vi "Stream.vi"(0 "reference in":refnum<class "Streamer.lvclass">, 5 "error in":errorcluster) -> (14 "reference out":refnum<class "Streamer.lvclass">, 19 "error out":errorcluster)   [LabVIEW 2023, in "Streamer.lvclass"]
uses:
  Streamer.lvclass
  <instrlib>/HPS-17000/HPS-17000.lvclass
  <vilib>/HPS-17000/MStream_grpc_CyclerMeasurement.ctl
  Streamer.lvclass/Streamer.ctl
  <vilib>/Utility/SystemLogging/NI_SystemLogging.lvlib
  <vilib>/HPS-17000/NI_BC_client.lvlib
panel:
  out "error info":errorcluster
  out "Last Command":string
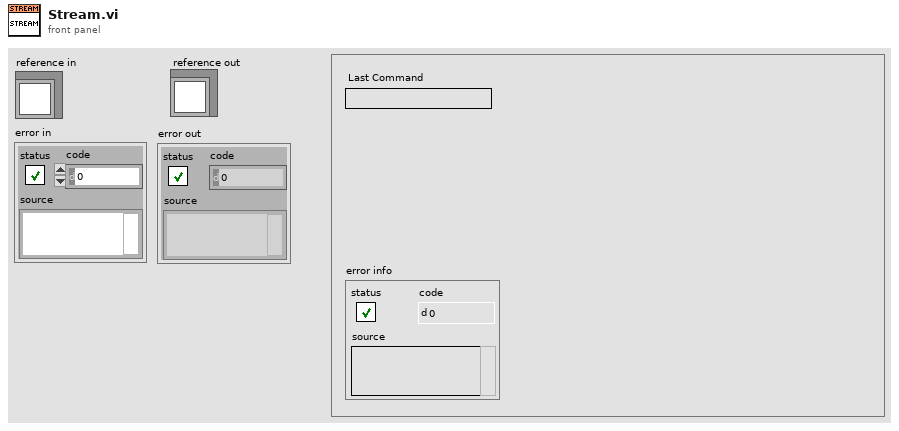
[diagram p1: front panel]
types:
  T1 = cluster{"Core":cluster{"Timeout":i32, "Events":cluster{"EventsToProcess":refnum<event-registration>}, "EventFromProcess":refnum<user-event>, "ProcessSyncQueue":refnum<queue>, "QueueFromProcess":refnum<queue>, "Command":string, "Data":variant}, "HPS17K Refs":refnum<class "HPS-17000.lvclass">[], "Stream Queues":refnum<queue>[]}
  T2 = enum32{"Invalid", "Standard", "Closed", "Hidden", "Minimized", "Maximized"}
  T3 = cluster{"EventsToProcess":refnum<event-registration>}
  T4 = typedef "NI_BC_client.lvlib/MStream_grpc_CyclerMeasurement.ctl" = cluster{"measured_voltage":sgl, "measured_current":sgl, "setpoint_voltage":sgl, "setpoint_current":sgl, "timestamp":i64}
  T5 = typedef "Streamer.lvclass/ObjectAttributes.ctl" = cluster{"HPS17K Refs":refnum<class "HPS-17000.lvclass">[], "Stream Queues":refnum<queue>[]}
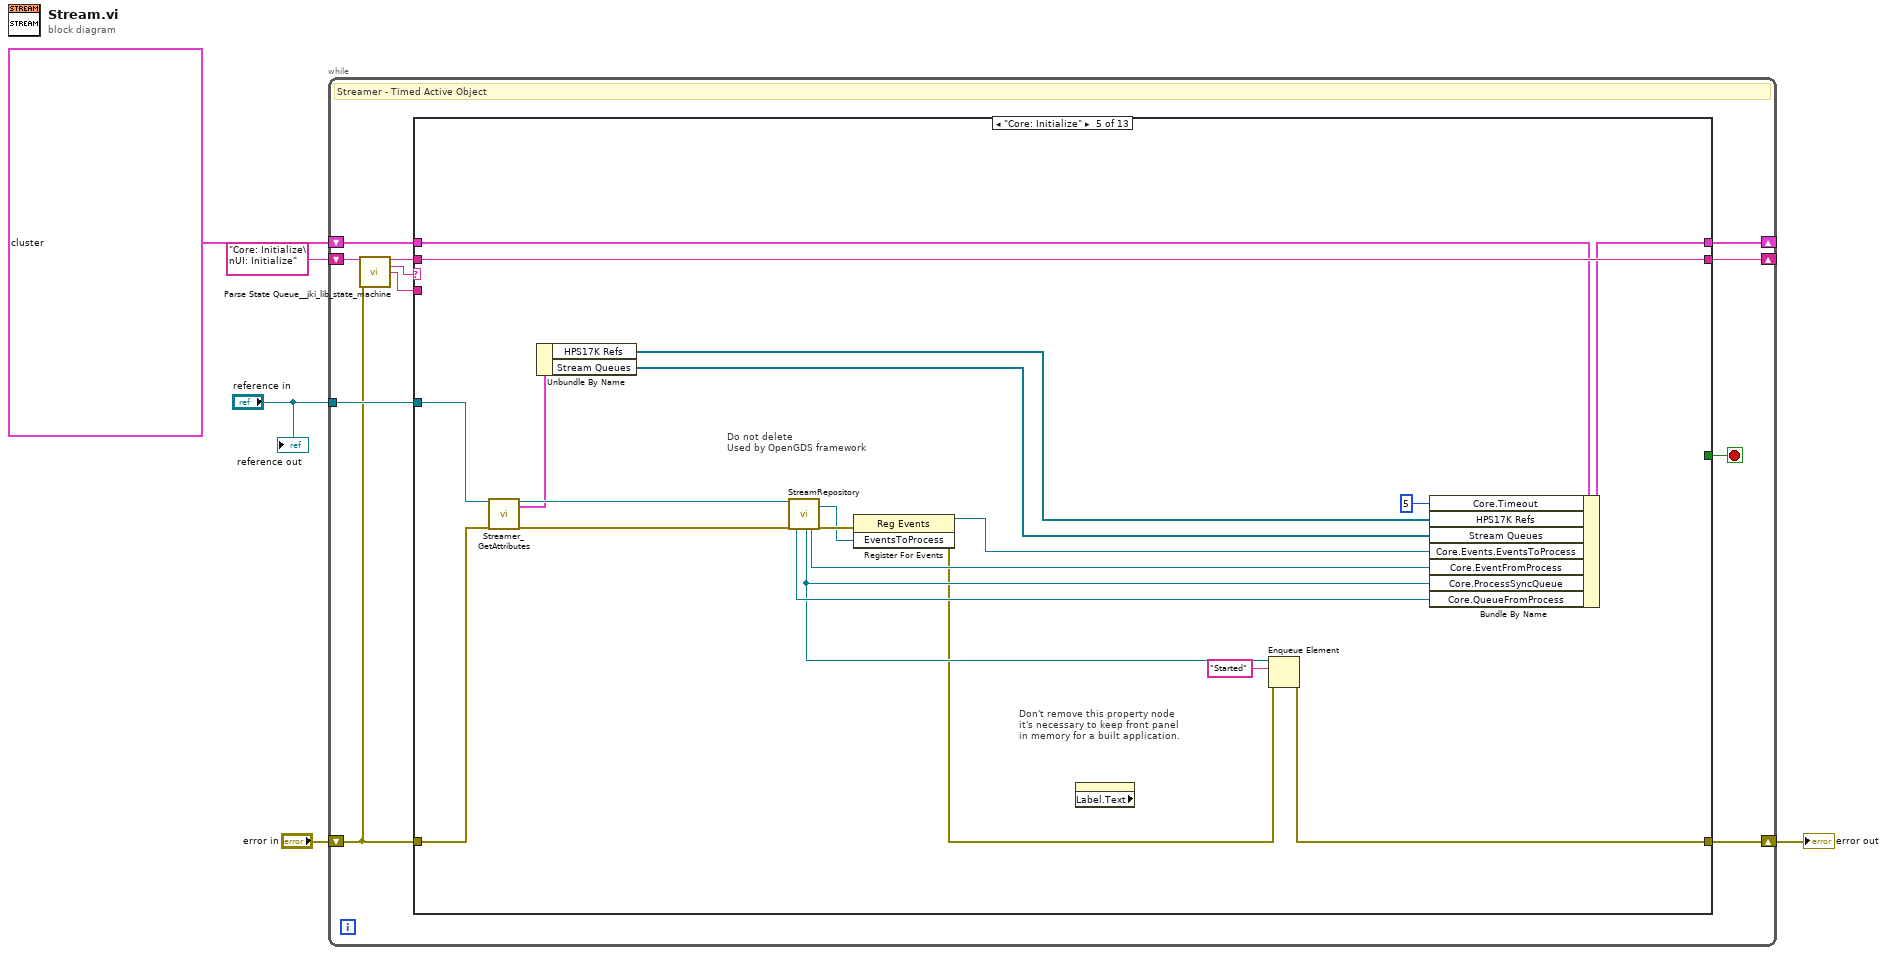
[diagram p0: block diagram]
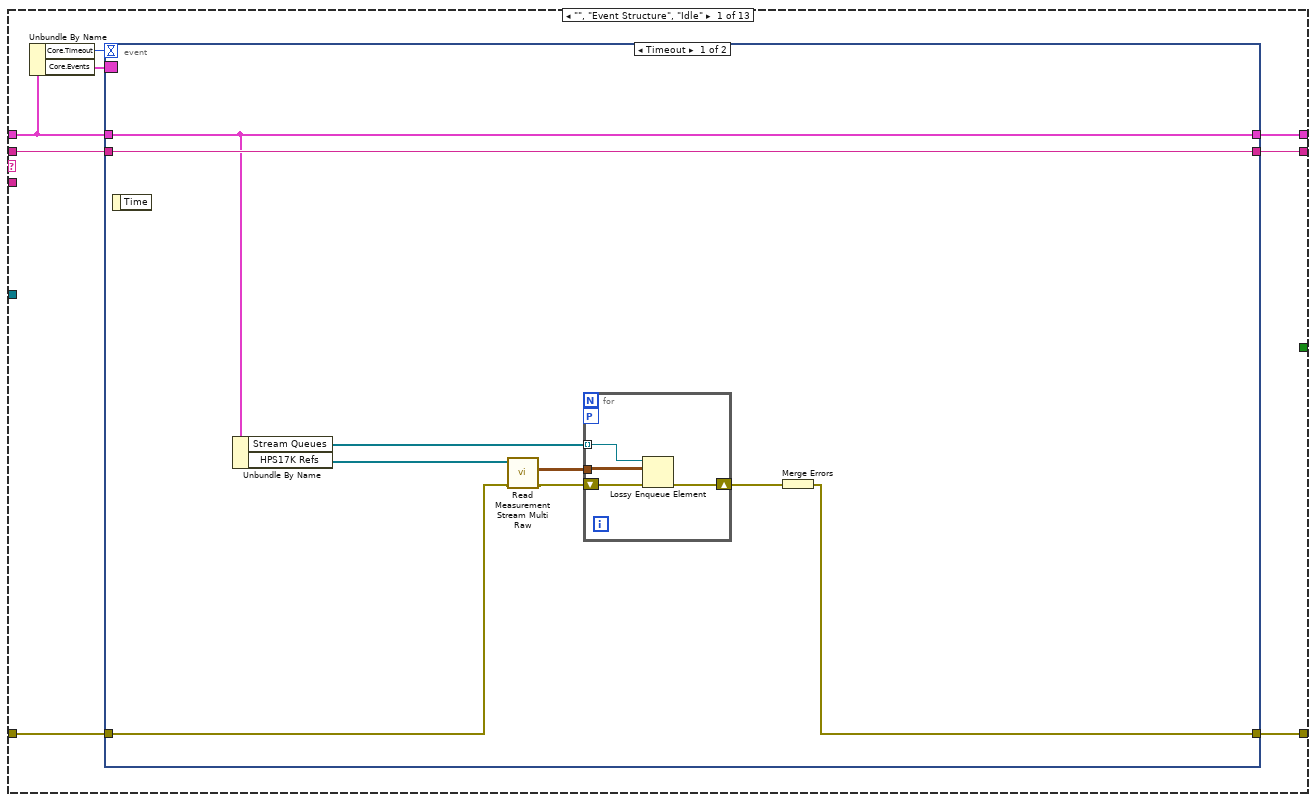
[diagram p2: hidden frame]
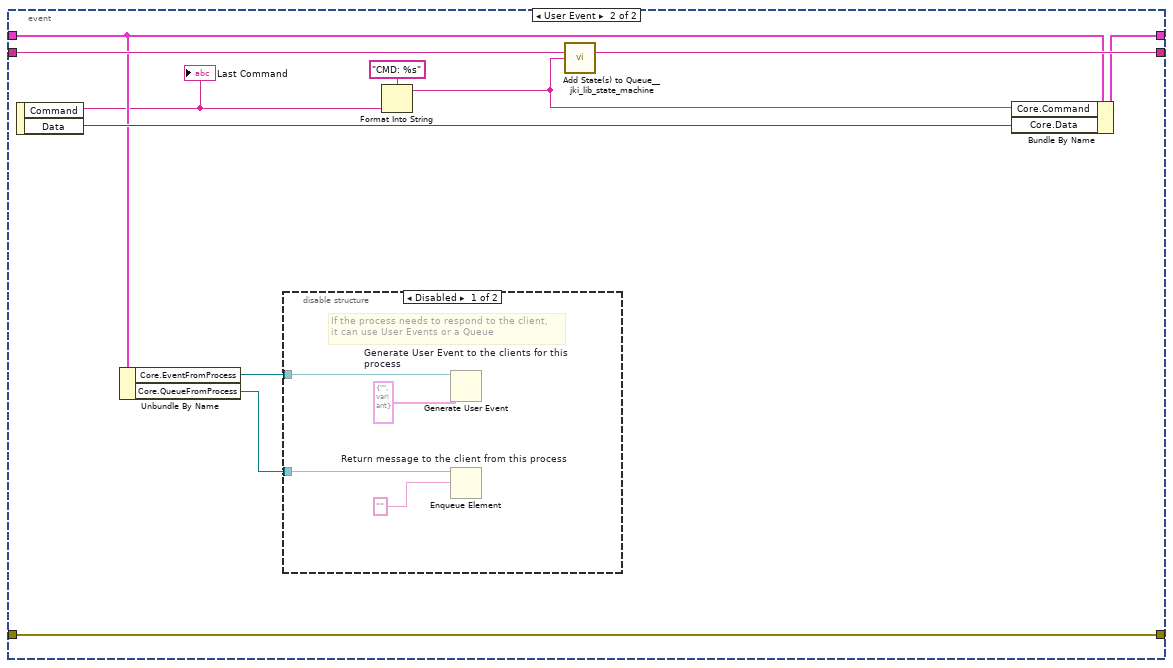
[diagram p3: hidden frame]
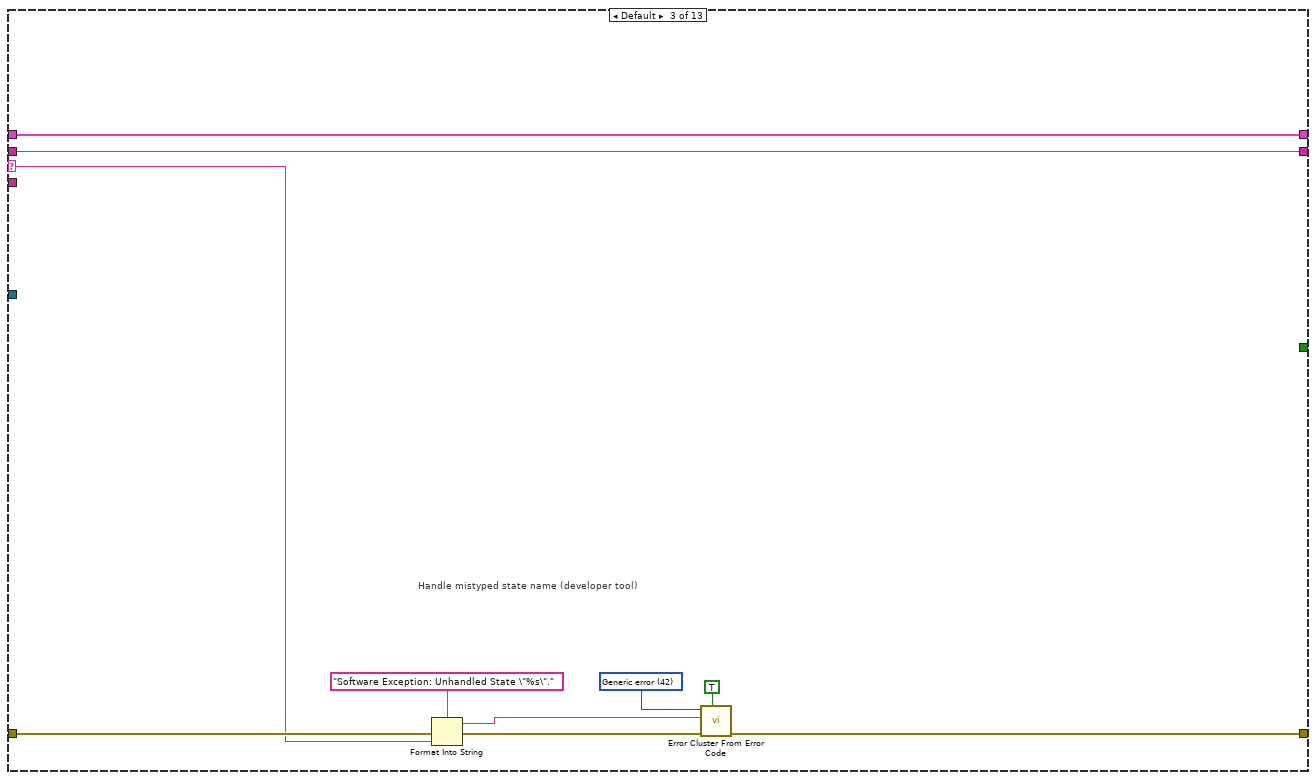
[diagram p6: hidden frame]
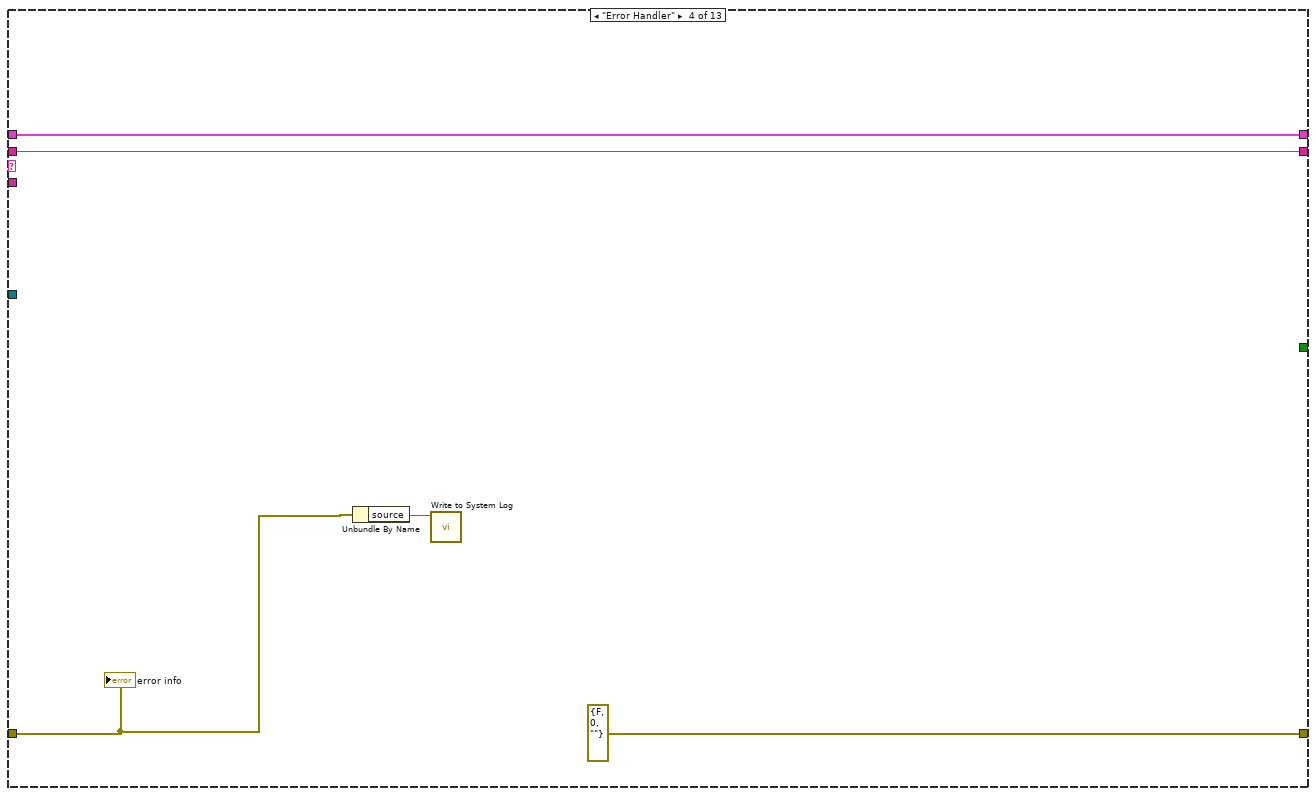
[diagram p7: hidden frame]
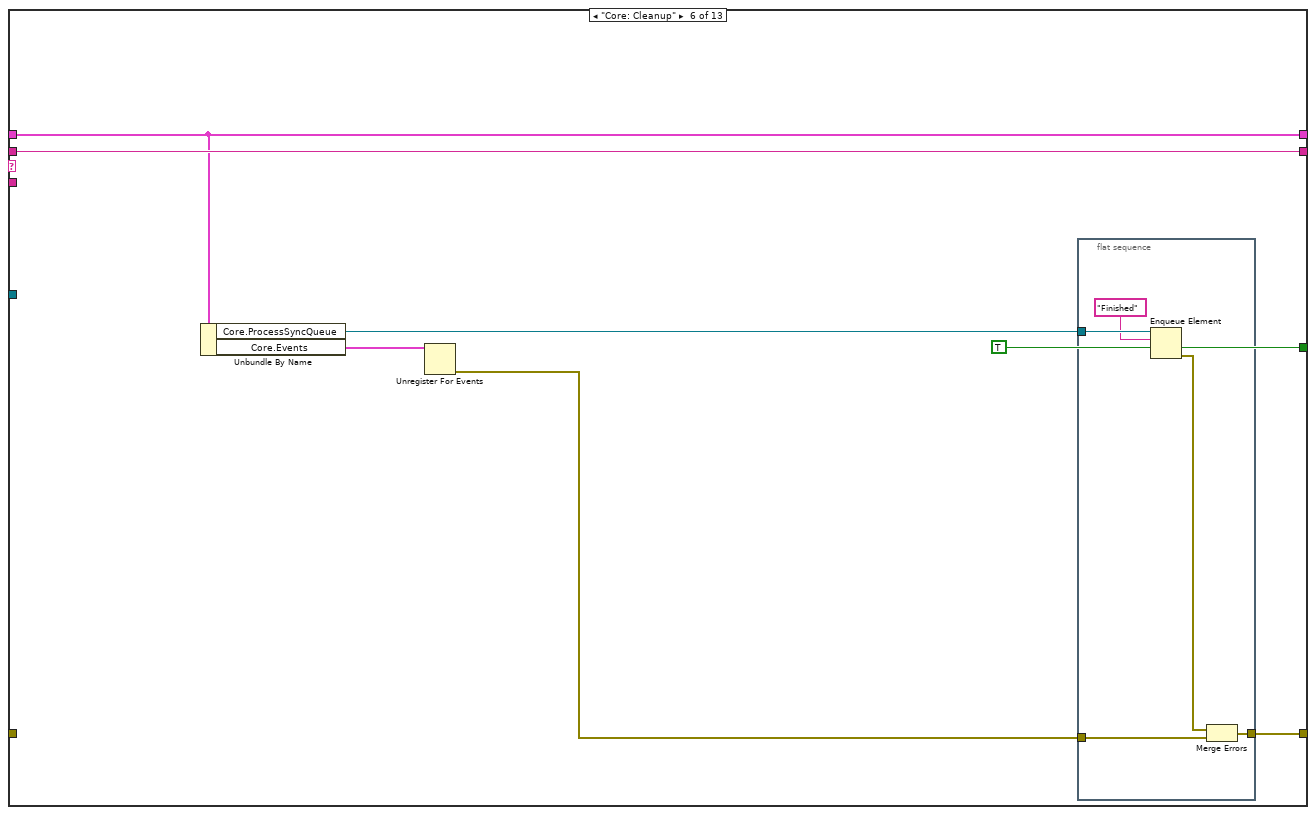
[diagram p8: hidden frame]
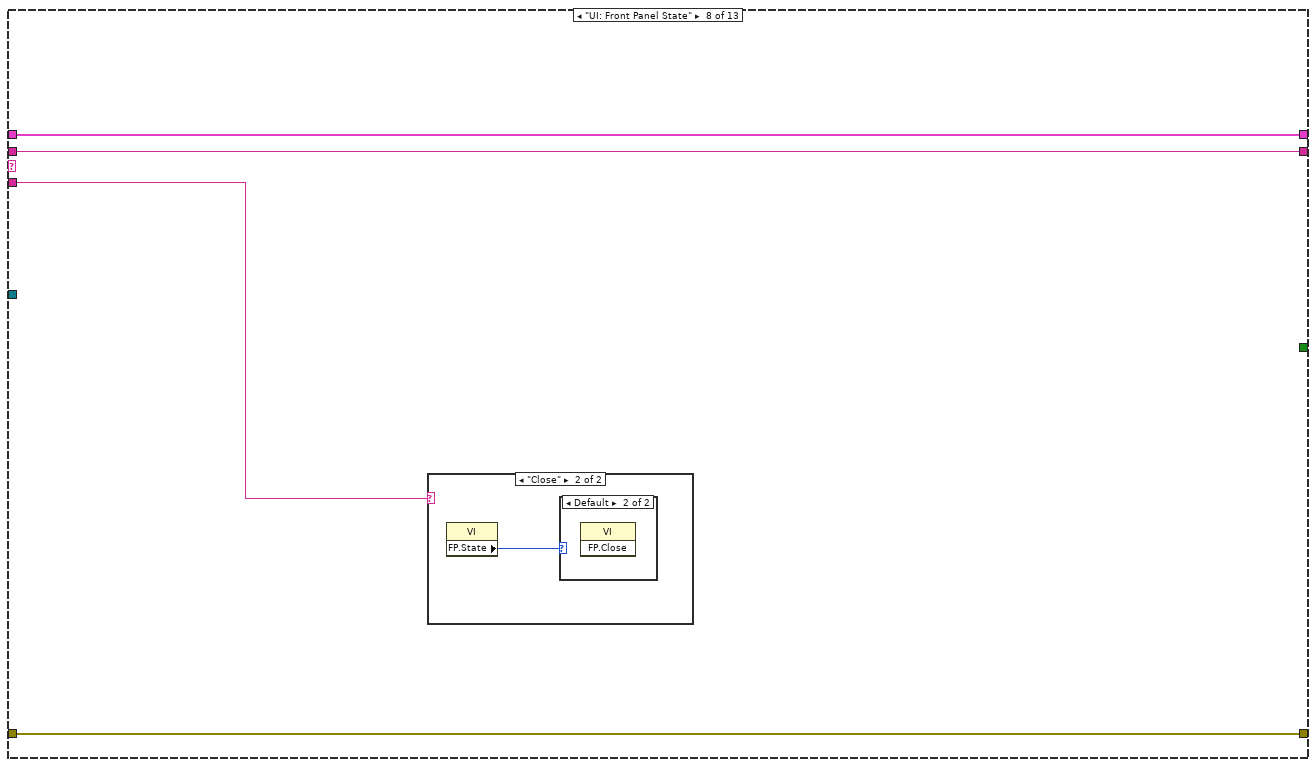
[diagram p10: hidden frame]
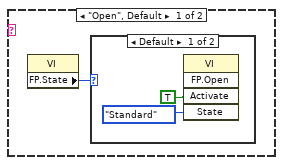
[diagram p11: hidden frame]
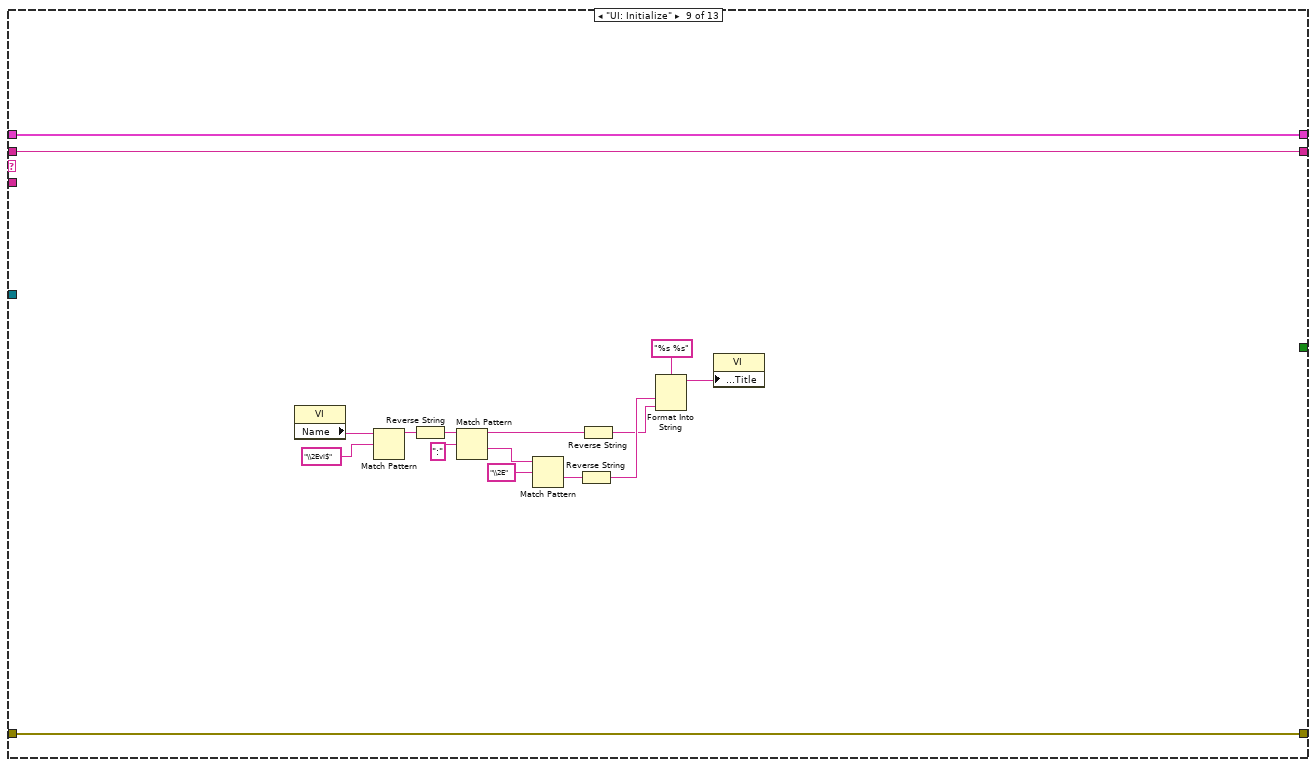
[diagram p14: hidden frame]
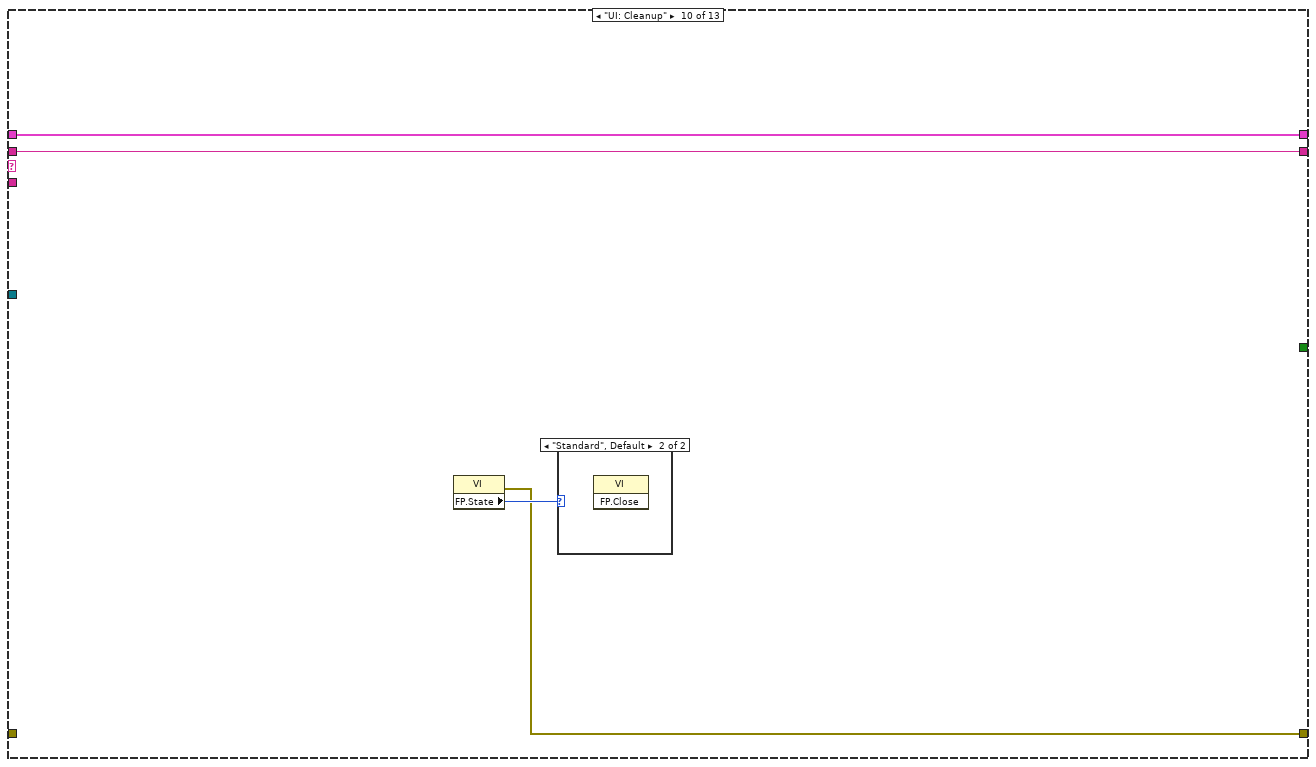
[diagram p15: hidden frame]
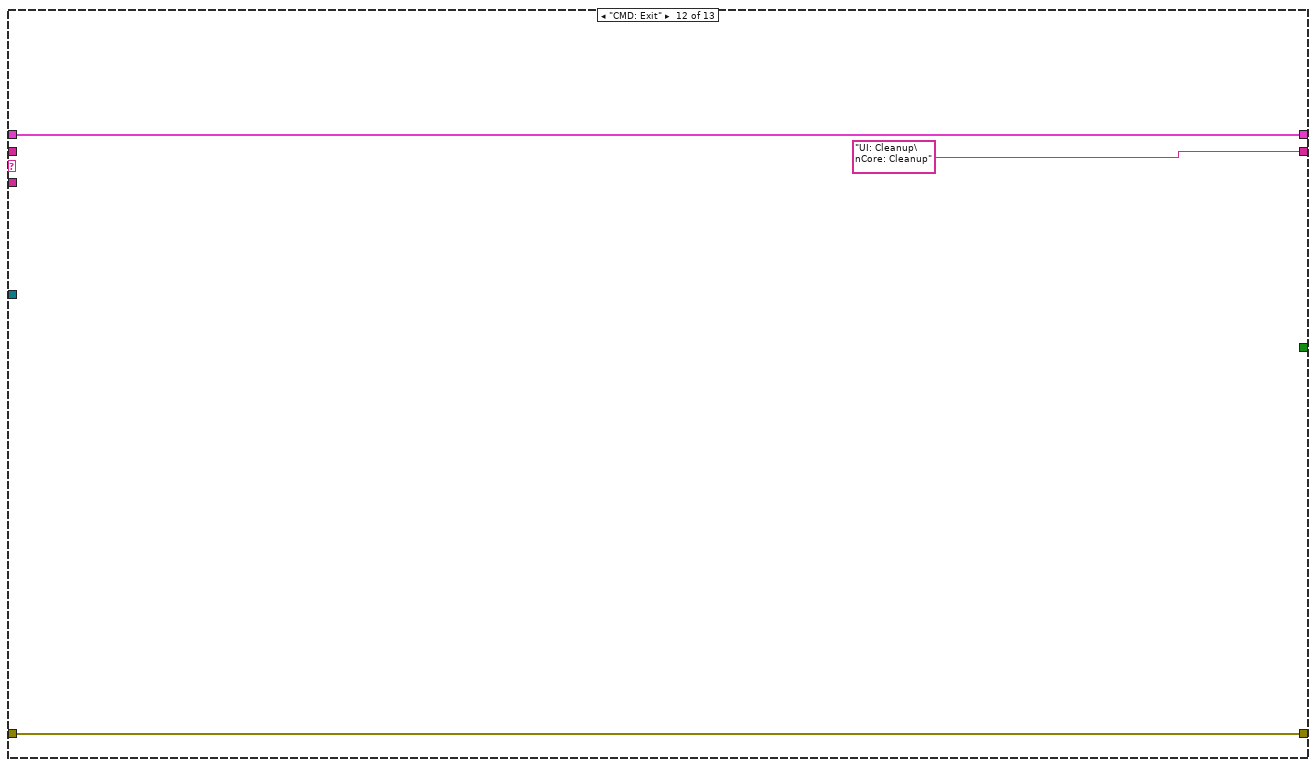
[diagram p18: hidden frame]
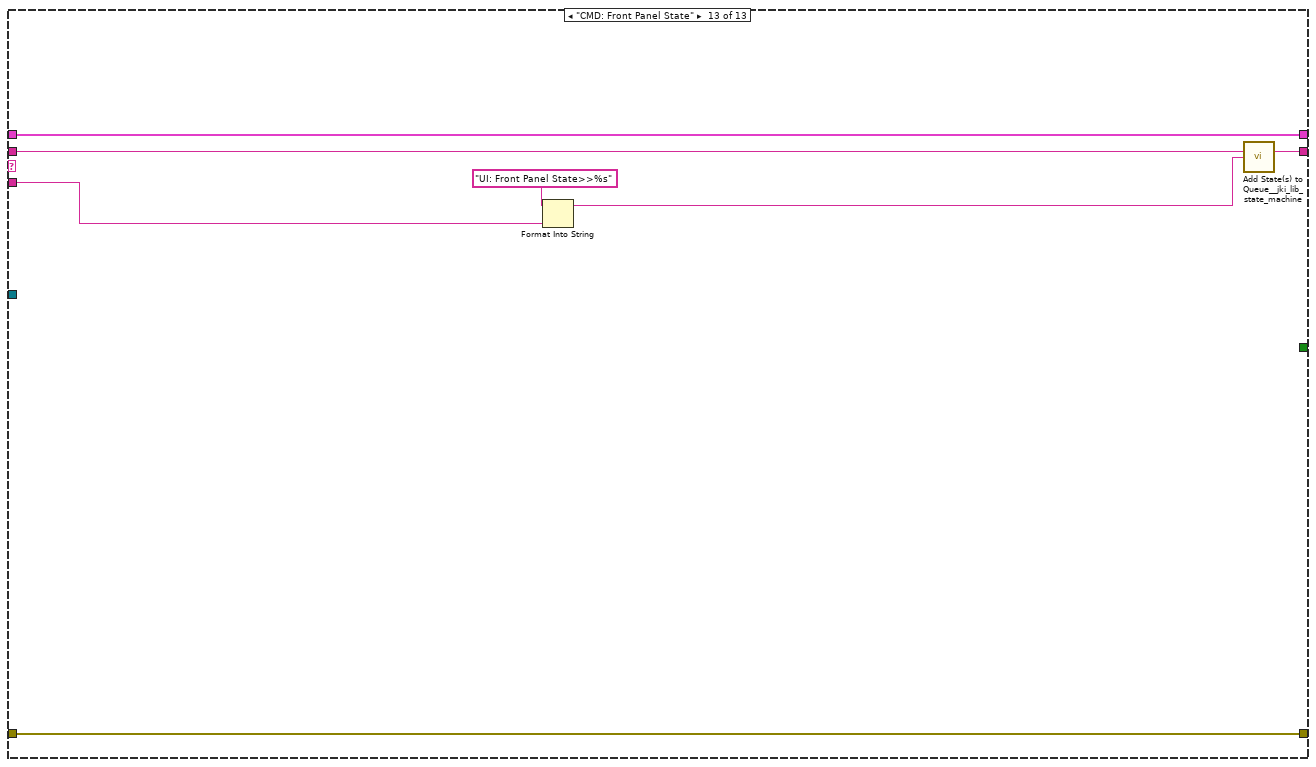
[diagram p19: hidden frame]
diagram:
  n1 = while {
    tunnel: "reference in" -> [w14]
    shift-right: [w13] -> _
    shift-left: T1 {"Core"={"Timeout"=-1, "Events"={"EventsToProcess"=refnum}, "EventFromProcess"=refnum, "ProcessSyncQueue"=refnum, "QueueFromProcess"=refnum, "Command"="", "Data"=variant}, "HPS17K Refs"=[], "Stream Queues"=[]} ("LocalVariables") -> [w16]
    shift-right: [w12] -> _
    shift-left: "Core: Initialize\nUI: Initialize" ("States Out") -> [w15]
    shift-right: [w7] -> w2
    shift-left: "error in" -> [w6]
    stop <- w8 stop-if-true
    # "Streamer - Timed Active Object"
    n2 = call <vilib>:"Parse State Queue__jki_lib_state_machine.vi"("State Queue"=w15, "Error In (no error)"=w6) -> ("Remaining States"=w10:string, "Current State"=w11:string, "Arguments"=w9:string)  [unwired: 11 in]
    n3 = case shown="\"Core: Initialize\"" w11 {
      selector: w11 -> [_ _ w56 _ _ _ _ _ _ _ _ _ _]
      tunnel: w6 -> [w18 w55 w58 w68 w75 _ w105 w106 w129 _ w136 w139 w146]
      tunnel: [w19 w55 w57 errorcluster {"status"=FALSE, "code"=0, "source"=""} ("error constant") w90 w93 w105 w106 w129 w130 w136 w139 w146] -> w7
      tunnel: [w24 w54 w65 w70 w88 w94 w104 w108 w122 w131 w135 w138 w145] -> w13
      tunnel: w16 -> [w20 w54 w65 w70 w87 w94 w104 w108 w122 w131 w135 w138 w145]
      tunnel: w10 -> [w22 w53 w64 w69 w89 w97 w103 w109 w114 w133 w134 _ w144]
      tunnel: w9 -> [_ _ _ _ _ _ _ w107 _ _ _ _ w141]
      tunnel: [w21 w53 w64 w69 w89 w97 w103 w109 w114 w133 w134 "UI: Cleanup\nCore: Cleanup" ("State(s) at Back (\"\")") w143] -> w12
      tunnel: [_ _ _ _ _ TRUE _ _ _ _ _ _ _] -> w8
      tunnel: w14 -> [_ _ _ _ w78 _ _ _ _ _ _ _ _]
      frame "", "Event Structure", "Idle" {
        n4 = Unbundle By Name(w20) -> ("Core.Timeout"=w17:i32, "Core.Events"=w23:T3)
        n5 = event shown="[0] Timeout" {
          selector: w23 -> [_ _]
          dyn-events: _ -> [_ _]
          timeout: w17 -> [_ _]
          tunnel: w20 -> [w30 w41]
          tunnel: [w30 w46] -> w24
          tunnel: [w33 w48] -> w21
          tunnel: w22 -> [w33 w47]
          tunnel: [w29 w42] -> w19
          tunnel: w18 -> [w28 w42]
          event Timeout {
            n6 = event-data() -> ()  [unwired: 1 in, 1 out]
            n7 = Unbundle By Name(w30) -> ("Stream Queues"=w32:refnum<queue>[], "HPS17K Refs"=w27:refnum<class "HPS-17000.lvclass">[])
            n8 = call <instrlib>:"Read Measurement Stream Multi Raw.vi"("error in"=w28, "cycler refs in"=w27) -> ("error out"=w26:errorcluster, "cycler measurements"=w25:T4[][])  [unwired: 7 in, 1 out]
            n9 = for {
              tunnel: w25 -> [w34]
              shift-right: [w36] -> w31
              shift-left: w26 -> [w37]
              tunnel: w32 -> [w35] mode=indexing
              workers-P: _ -> [_]
              n10 = Lossy Enqueue Element(queue=w35, element=w34, error in (no error)=w37) -> (error out=w36:errorcluster)  [unwired: 3 out]
            }
            n11 = Merge Errors(w31) -> (w29:errorcluster)
          }
          event User Event {
            n12 = event-data() -> ("Command"=w39:string, "Data"=w45:variant)  [unwired: 1 in]
            "Last Command" <- w39
            n13 = Unbundle By Name(w41) -> ("Core.EventFromProcess"=w44:refnum<user-event>, "Core.QueueFromProcess"=w43:refnum<queue>)
            n14 = disable-structure shown="Disabled" {
              disable-tunnel: w44 -> [w52 _]
              disable-tunnel: w43 -> [w51 _]
              frame Disabled {
                # "If the process needs to respond to the client,\nit can use User Events or a Queue"
                n15 = Generate User Event "Generate User Event to the clients for this process"(user event=w52, event data cluster=cluster{"Command":string, "Data":variant} {"Command"="", "Data"=variant} ("event data")) -> ()  [unwired: 2 in, 2 out]
                n16 = Enqueue Element "Return message to the client from this process"(queue=w51, element="") -> ()  [unwired: 2 in, 3 out]
              }
              frame Enabled {
              }
            }
            n17 = Format Into String(format string="CMD: %s", w39) -> (resulting string=w38:string)  [unwired: 2 in, 1 out]
            n18 = call <vilib>:"Add State(s) to Queue__jki_lib_state_machine.vi"("State(s) in (\"\")"=w47, "State(s) at Back (\"\")"=w38) -> ("States Out"=w48:string)  [unwired: 13 in]
            n19 = Bundle By Name(cluster=w41, "Core.Command"=w38, "Core.Data"=w45) -> (w46:T1)
          }
        }
      }
      frame "---------- Core ----------" {
      }
      frame Default {
        w62 = 42 items=["No error", "Argument error", "Memory is full", "Out of zone", "End of file", "File already open", "Generic file I/O error", "File not found", "File permission error", "Disk is full", "Duplicate path", "Too many files open", "System feature not enabled", "Resource file not found", "Cannot add resource", "Resource not found", "Image not found", "Image memory error", "Pen does not exist", "Config type invalid", "Config token not found", "Config parse error", "Config memory error", "Bad external code format", "Bad external code offset", "External code not present", "Null window", "Destroy window error", "Null menu", "Print aborted", "Bad print record", "Print driver error", "Windows error during printing", "Memory error during printing", "Print dialog error", "Generic print error", "Invalid device refnum", "Device not found", "Device parameter error", "Device unit error", "Cannot open device", "Device call aborted", "Generic error", "Cancelled by user", "Object ID too low", "Object ID too high", "Object not in heap", "Unknown heap", "Unknown object (invalid DefProc)", "Unknown object (DefProc not in table)", "Message out of range", "Invalid (null) method", "Unknown message", "Manager call not supported", "Bad address", "Network operation in progress", "Network operation timed out", "Connection is busy", "Network attribute not supported", "Network error", "Address in use", "System out of memory", "Connection aborted", "Connection refused", "Not connected", "Already connected", "Connection closed", "Initialization error (interapplication manager)", "Bad occurrence", "Wait on unbound occurrence handler", "Occurrence queue overflow", "Datalog type conflict", "Unused", "Unrecognized type (interapplication manager)", "Memory corrupt", "Failed to make temporary DLL", "Old CIN version", "Drag socket not found", "Failed to load drop-object", "Failed to register OLE object", "Failed to release OLE object", "Format specifier type mismatch", "Unknown format specifier", "Too few format specifiers", "Too many format specifiers", "Scan failed", "Newer CIN version", "Error converting to variant", "Runtime menu error", "Password tampered", "Variant attribute not found", "Incompatible variant data type", "Event data is not available", "Event Store is not present", "Occurrence is not found", "Event Queue is not created", "Event info is not available", "Refnum passed is NULL", "Error retrieving Class GUID", "Error retrieving CoClass GUID", "Error retrieving TypeLib GUID.", "Bad built application magic bytes.", "Specific driver is different from the specific driver associated with the Logical Name.", "There is no session opened to the class driver.", "Max Error", "MAX - Error with config objects", "MAX - Error loading configuration", "MAX - Group not supported"]
        # "Handle mistyped state name (developer tool)"
        n20 = Format Into String(format string="Software Exception: Unhandled State \"%s\"." ("message"), error in=w58, w56) -> (resulting string=w61:string, error out=w60:errorcluster)  [unwired: 1 in]
        n21 = call <vilib>:"Error Cluster From Error Code.vi"("show call chain? (False)"=TRUE, "error in (no error)"=w60, "error message (\"\")"=w61, "error code (0)"=w62) -> ("error out"=w57:errorcluster)  [unwired: 5 in]
      }
      frame "Error Handler" {
        n22 = Unbundle By Name(w68) -> ("source"=w66:string)
        n23 = call <vilib>:"Write to System Log.vi"("message"=w66) -> ()  [unwired: 10 in, 1 out]
        "error info" <- w68
      }
      frame "Core: Initialize" {
        # "Do not delete\nUsed by OpenGDS framework"
        # "Don't remove this property node\nit's necessary to keep front panel\nin memory for a built application."
        # "Template created by VI Technologies"
        n24 = call "Streamer_GetAttributes.vi"("reference in"=w78, "Error In"=w75) -> ("reference out"=w77:refnum<class "Streamer.lvclass">, "Data"=w74:T5, "Error Out"=w76:errorcluster)  [unwired: 14 in, 1 out]
        n25 = Unbundle By Name(w74) -> ("HPS17K Refs"=w73:refnum<class "HPS-17000.lvclass">[], "Stream Queues"=w72:refnum<queue>[])
        n26 = call "StreamRepository.vi"("reference in"=w77, "Error In"=w76) -> ("QueueFromProcess"=w82:refnum<queue>, "ProcessSyncQueue"=w80:refnum<queue>, "EventFromProcess"=w83:refnum<user-event>, "EventsToProcess"=w85:refnum<user-event>, "Error Out"=w86:errorcluster)  [unwired: 10 in, 3 out]
        n27 = register-events(error in=w86, w85) -> (reference out=w84:refnum<event-registration>, error out=w79:errorcluster)  [unwired: 1 in]
        n28 = property on="reference in" class="LVClassControl (strict)" props=["Label", "Text"]() -> ()  [unwired: 2 in, 3 out]
        n29 = Enqueue Element(queue=w80, element="Started", error in (no error)=w79) -> (error out=w90:errorcluster)  [unwired: 1 in, 2 out]
        n30 = Bundle By Name(cluster=w87, "Core.Timeout"=5, "HPS17K Refs"=w73, "Stream Queues"=w72, "Core.Events.EventsToProcess"=w84, "Core.EventFromProcess"=w83, "Core.ProcessSyncQueue"=w80, "Core.QueueFromProcess"=w82) -> (w88:T1)
      }
      frame "Core: Cleanup" {
        n31 = Unbundle By Name(w94) -> ("Core.ProcessSyncQueue"=w95:refnum<queue>, "Core.Events"=w92:T3)
        n32 = Unregister For Events(event registration refnum=w92) -> (error out=w91:errorcluster)  [unwired: 1 in]
        n33 = flat-sequence {
          tunnel: [w101] -> w93
          tunnel: w95 -> [w100]
          tunnel: w91 -> [w99]
          frame #0 {
            n34 = Enqueue Element(queue=w100, element="Finished") -> (error out=w102:errorcluster)  [unwired: 2 in, 2 out]
            n35 = Merge Errors(w102, w99) -> (w101:errorcluster)
          }
        }
      }
      frame "---------- UI ----------" {
      }
      frame "UI: Front Panel State" {
        n36 = case shown="\"Close\"" w107 {
          frame "Open", Default {
            n37 = property class="VI"() -> ("FP.State"=w110:T2)  [unwired: 2 in, 2 out]
            n38 = case shown="Default" w110 {
              frame Default {
                n39 = invoke class="VI" method="FP.Open"("Activate"=TRUE, "State"=T2."Standard") -> ()  [unwired: 3 in, 5 out]
              }
              frame "Standard" {
              }
            }
          }
          frame "Close" {
            n40 = property class="VI"() -> ("FP.State"=w113:T2)  [unwired: 2 in, 2 out]
            n41 = case shown="Default" w113 {
              frame "Closed" {
              }
              frame Default {
                n42 = invoke class="VI" method="FP.Close"() -> ()  [unwired: 3 in, 3 out]
              }
            }
          }
        }
      }
      frame "UI: Initialize" {
        n43 = property class="VI"() -> ("Name"=w128:string)  [unwired: 2 in, 2 out]
        n44 = Match Pattern(string=w128, regular expression="\\2Evi$") -> (before substring=w126:string)  [unwired: 1 in, 3 out]
        n45 = Reverse String(1:w126) -> (0:w125:string)
        n46 = Match Pattern(string=w125, regular expression=":") -> (before substring=w123:string, after substring=w121:string)  [unwired: 1 in, 2 out]
        n47 = Match Pattern(string=w121, regular expression="\\2E") -> (after substring=w119:string)  [unwired: 1 in, 3 out]
        n48 = Reverse String(1:w119) -> (0:w118:string)
        n49 = Reverse String(1:w123) -> (0:w117:string)
        n50 = Format Into String(format string="%s %s", w118, w117) -> (resulting string=w116:string)  [unwired: 2 in, 1 out]
        n51 = property class="VI"("Front Panel.Title"=w116) -> ()  [unwired: 2 in, 2 out]
      }
      frame "UI: Cleanup" {
        n52 = property class="VI"() -> (error out=w130:errorcluster, "FP.State"=w132:T2)  [unwired: 2 in, 1 out]
        n53 = case shown="\"Standard\", Default" w132 {
          frame "Closed" {
          }
          frame "Standard", Default {
            n54 = invoke class="VI" method="FP.Close"() -> ()  [unwired: 3 in, 3 out]
          }
        }
      }
      frame "---------- CMD ----------" {
      }
      frame "CMD: Exit" {
      }
      frame "CMD: Front Panel State" {
        n55 = Format Into String(format string="UI: Front Panel State>>%s" ("string"), w141) -> (resulting string=w140:string)  [unwired: 2 in, 1 out]
        n56 = call <vilib>:"Add State(s) to Queue__jki_lib_state_machine.vi"("State(s) in (\"\")"=w144, "State(s) at Back (\"\")"=w140) -> ("States Out"=w143:string)  [unwired: 13 in]
      }
    }
  }
  "error out" <- w2
  "reference out" <- "reference in"
